vi "GetSingleCalibr.vi"(8 "error in (no error)":errorcluster, 10 "ID":string, 11 "ByteGSWebAPI-V0 in":refnum<class "ByteGSWebAPI-V0.lvclass">) -> (0 "error out":errorcluster, 2 "CalibrationData":T1, 3 "ByteGSWebAPI-V0 out":refnum<class "ByteGSWebAPI-V0.lvclass">, 4 "body":string, 6 "headers":string)   [LabVIEW 2019, in "ByteGSWebAPI.lvlib" / "ByteGSWebAPI-V0.lvclass"]
uses:
  ByteGSWebAPI-V0.lvclass
  Cntrls/SingleCalibration.ctl
  54c15d21-1fd3-4ea8-80e2-c69b0da6434b.vi
  <vilib>/JDP Science/JSONtext/JSON text to Variant.vi
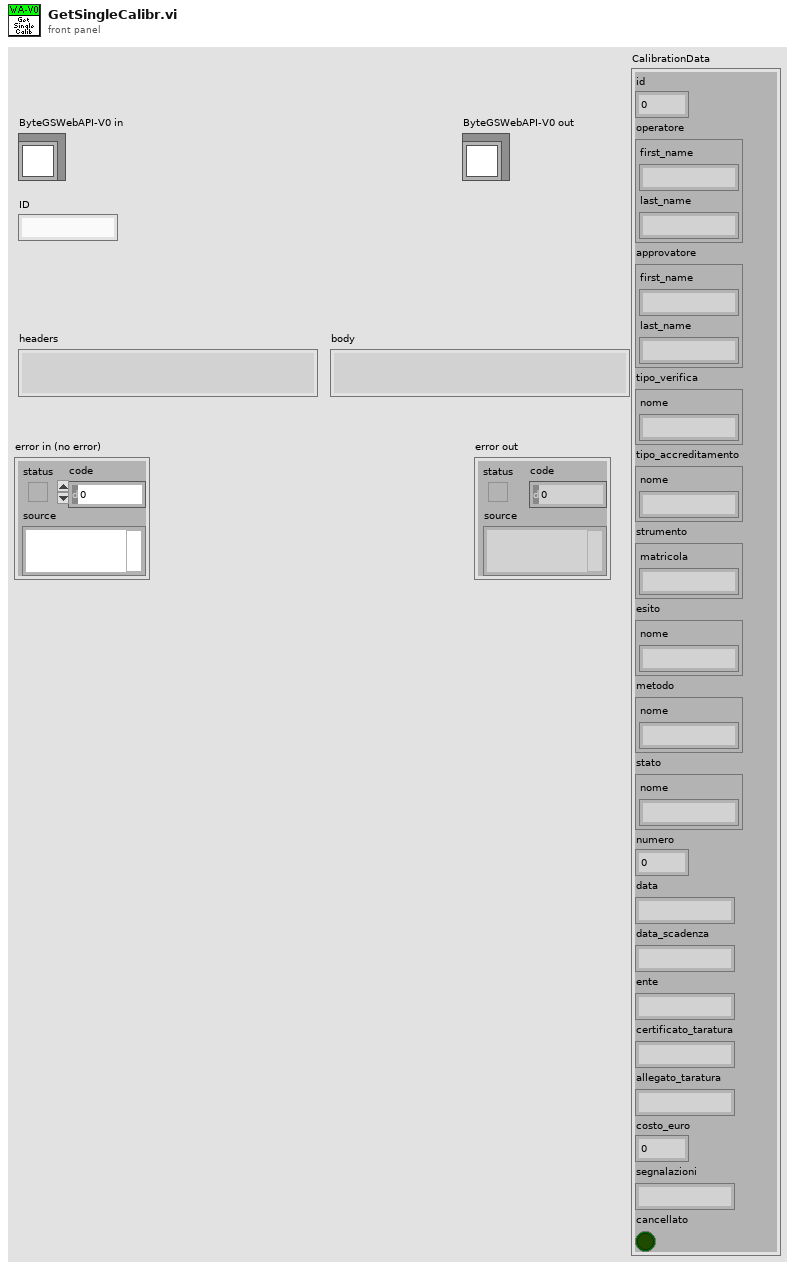
[diagram p1: front panel]
types:
  T1 = typedef "ByteGSWebAPI.lvlib/ByteGSWebAPI-V0.lvclass/SingleCalibration.ctl" = cluster{"id":i32, "operatore":cluster{"first_name":string, "last_name":string}, "approvatore":cluster{"first_name":string, "last_name":string}, "tipo_verifica":cluster{"nome":string}, "tipo_accreditamento":cluster{"nome":string}, "strumento":cluster{"matricola":string}, "esito":cluster{"nome":string}, "metodo":cluster{"nome":string}, "stato":cluster{"nome":string}, "numero":i32, "data":string, "data_scadenza":string, "ente":string, "certificato_taratura":string, "allegato_taratura":string, "costo_euro":dbl, "segnalazioni":string, "cancellato":bool}
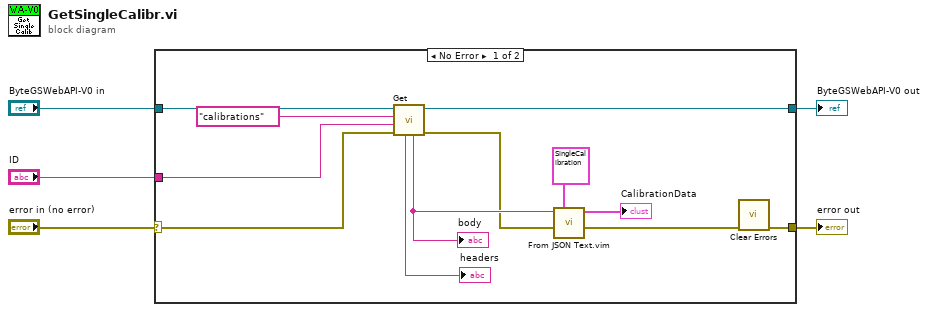
[diagram p0: block diagram]
diagram:
  n1 = case shown="No Error" "error in (no error)" {
    selector: "error in (no error)" -> [w14 w19]
    tunnel: [w8 w19] -> w4
    tunnel: [w16 w18] -> w2
    tunnel: "ByteGSWebAPI-V0 in" -> [w17 w18]
    tunnel: "ID" -> [w12 _]
    frame No Error {
      n2 = call-dynamic "Get.vi"("error in (no error)"=w14, "Parameter"=w12, "Request"="calibrations" ("Parameter"), "ByteGSWebAPI-V0 in"=w17) -> ("error out"=w10:errorcluster, "ByteGSWebAPI-V0 out"=w16:refnum<class "ByteGSWebAPI-V0.lvclass">, "body"=w11:string, "headers"=→"headers":string)  [unwired: 4 in]
      "body" <- w11
      n3 = call "From JSON Text.vim"("Data Type and Default Value"=T1 {"id"=0, "operatore"={"first_name"="", "last_name"=""}, "approvatore"={"first_name"="", "last_name"=""}, "tipo_verifica"={"nome"=""}, "tipo_accreditamento"={"nome"=""}, "strumento"={"matricola"=""}, "esito"={"nome"=""}, "metodo"={"nome"=""}, "stato"={"nome"=""}, "numero"=0, "data"="", "data_scadenza"="", "ente"="", "certificato_taratura"="", "allegato_taratura"="", "costo_euro"=0.0, "segnalazioni"="", "cancellato"=FALSE} ("Calibration"), "error in (no error)"=w10, "JSON"=w11) -> ("error out"=w9:errorcluster, "Data out"=→"CalibrationData":T1)  [unwired: 7 in]
      n4 = call <vilib>:"Clear Errors.vi"("error in (no error)"=w9) -> ("error out"=w8:errorcluster)  [unwired: 5 in, 1 out]
    }
    frame Error {
    }
  }
  "error out" <- w4
  "ByteGSWebAPI-V0 out" <- w2
